vi "Module Information.vi"(7 "Module Name":string="Module") -> ()   [LabVIEW 2017, in "DebugConsole.lvlib"]
uses:
  DebugConsole.lvlib
  _Support/Typedef/_CSM_MODE.ctl
  _Support/CSMQ/_CSMOFGVOPER.ctl
  _csmlite/_PassAllowedMessage - MsgList.vi
  _csmlite/_csmlite.lvlib
  Communicable State Machine.lvlib
  _ui/csm-ui-support.lvlib
panel:
  in  "CSM":string
  out "#Nodes":i32
  out "Mode":T1=enum."Stand Alone"
  out "inlvlibp":bool
  out "interStop":bool
  out "#Elements In Queue":i32
  out "Initialized":enum16{"Initializing", "Ready", "Exiting"}(ring)
  out "RemoteMessge?":bool
  out "Current State":string
  out "Remaing States":string
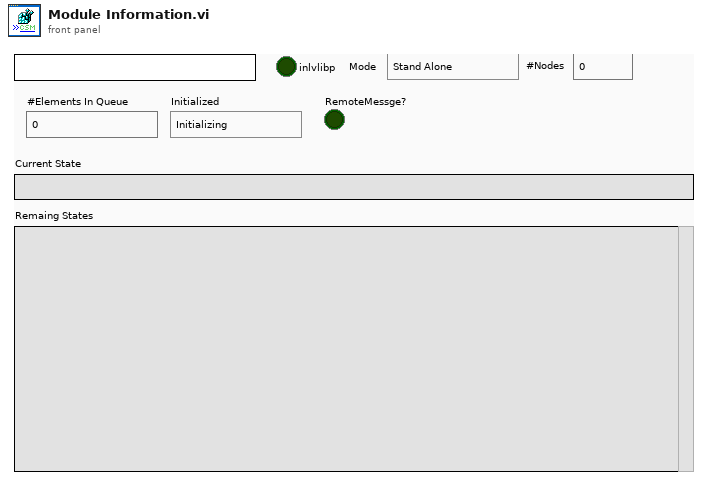
[diagram p1: front panel]
types:
  T1 = typedef "Communicable State Machine.lvlib/_CSM_MODE.ctl" = enum16{"Not Exist", "Stand Alone", "CSM", "Worker", "Worker Agent", "Chain Node", "Chain"}
  T2 = enum32{"Invalid", "Standard", "Closed", "Hidden", "Minimized", "Maximized"}
  T3 = enum32{"invalid app kind", "Development System", "Run Time System", "Student Edition", "Embedded LabVIEW", "Evaluation", "Custom"}
  T4 = cluster{"Core":cluster{"Current VI Reference":refnum<vi>, "Close Panel on Exit?":bool}, "Your Boolean data":bool, "Your string data":string}
  T5 = cluster{"Current VI Reference":refnum<vi>, "Close Panel on Exit?":bool}
  T6 = typedef "Communicable State Machine.lvlib/_CSMOFGVOPER.ctl" = enum16{"Create If not Exist", "Get By Name", "List", "Check If Name Exists", "Release", "Module Status", "Create Status Event Handler", "Destroy Status Event Handler", "Clear Invalid Objs"}
  T7 = enum8{"Enabled", "Disabled", "Disabled and Grayed Out"}
  T8 = typedef "Communicable State Machine.lvlib/_CSMObj.ctl" = cluster{"info":T9, "Refs":T10}
  T9 = typedef "Communicable State Machine.lvlib/_CSMObj-Info.ctl" = cluster{"Module Name":string, "Requested Name":string, "Group Name":string, "Mode":T1, "Allowed Messages":string[]}
  T10 = typedef "Communicable State Machine.lvlib/_CSMObj-Refs.ctl" = cluster{"WatchDogQ":refnum<queue>, "CSMDataDVR":refnum<data-value>, "Queue":T11, "GroupDataDVR":refnum<data-value>, "TagMap":refnum<data-value>, "ExitEvent":refnum<user-event>, "NewStateEvent":refnum<user-event>, "StatusEvent":refnum<user-event>, "InterruptEvent":refnum<user-event>}
  T11 = typedef "Communicable State Machine.lvlib/Priority Queue.ctl" = cluster{"HPriorityQ":refnum<queue>, "LowPriorityQ":refnum<queue>}
  T12 = typedef "Communicable State Machine.lvlib/_CSMObj-Data.ctl" = cluster{"RemoteMessge?":bool, "error":errorcluster, "Return State":string, "Initialized":enum16{"Initializing", "Ready", "Exiting"}, "InternalRegistryRules":string[], "Return Msg Type":T13, "Current State":string, "Remaing JKISM Queue":string}
  T13 = typedef "Communicable State Machine.lvlib/_CSM_MSG_TYPE.ctl" = enum16{"Sync Message(-@)", "Async Message(->)", "Async without Response(->|)", "Async Response", "Broadcast(-><all>)", "Broadcast(-><status>)", "Broadcast(-><interrupt>)", "Append to JKISM States", "Append to JKISM States(High Priority)", "Broadcast(-><state>)", "<None>"}
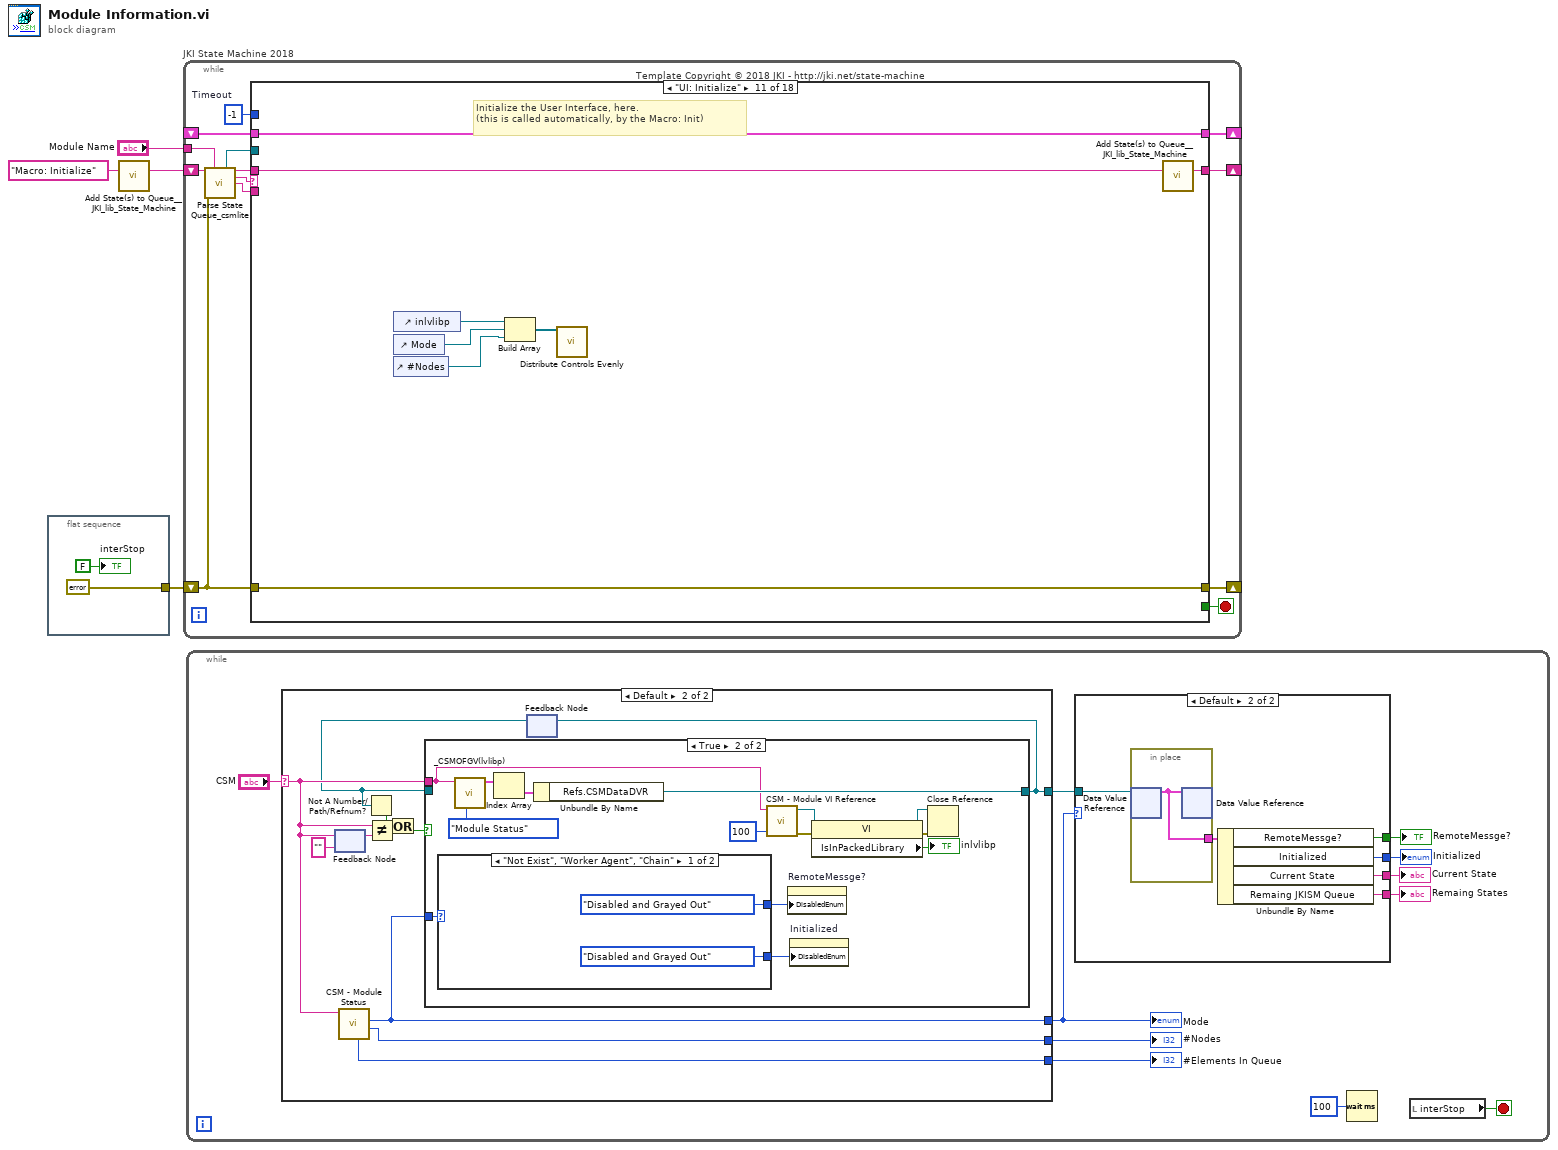
[diagram p0: block diagram]
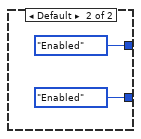
[diagram p5: hidden frame]
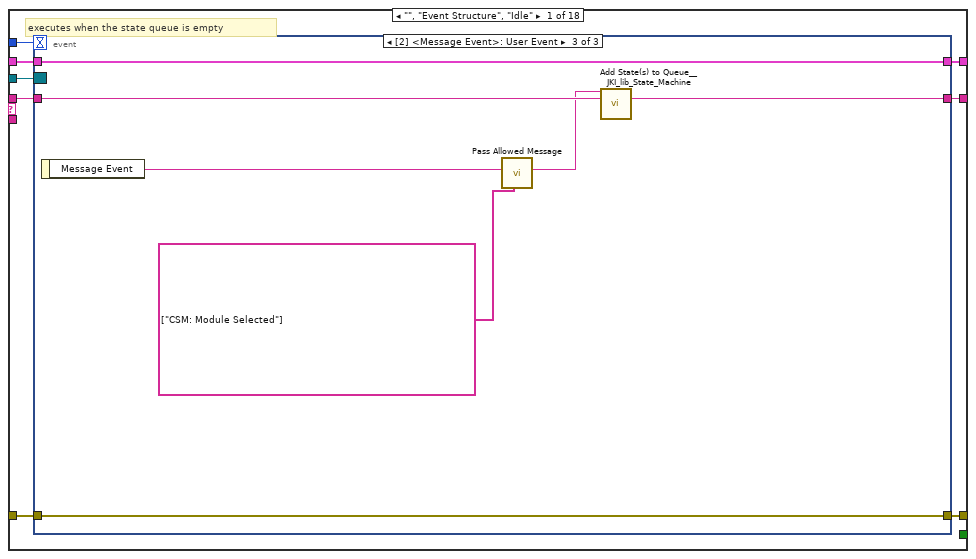
[diagram p6: hidden frame]
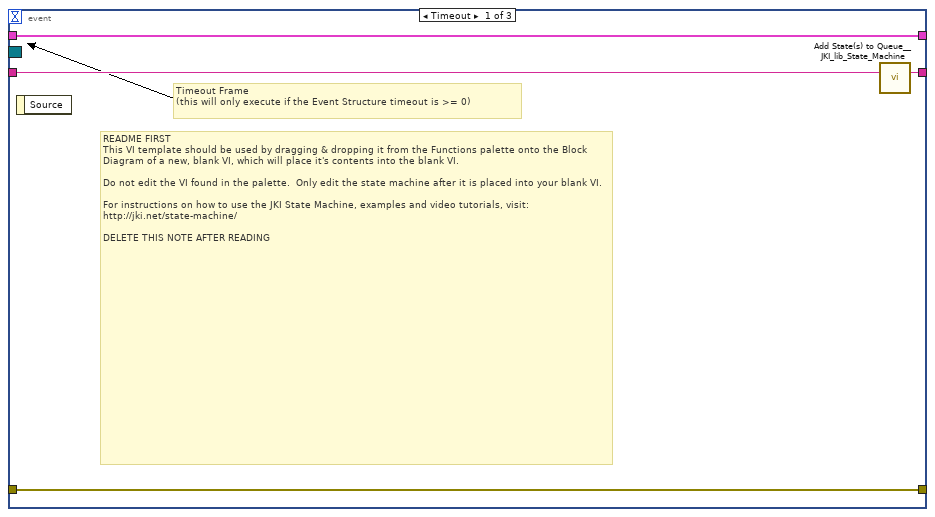
[diagram p7: hidden frame]
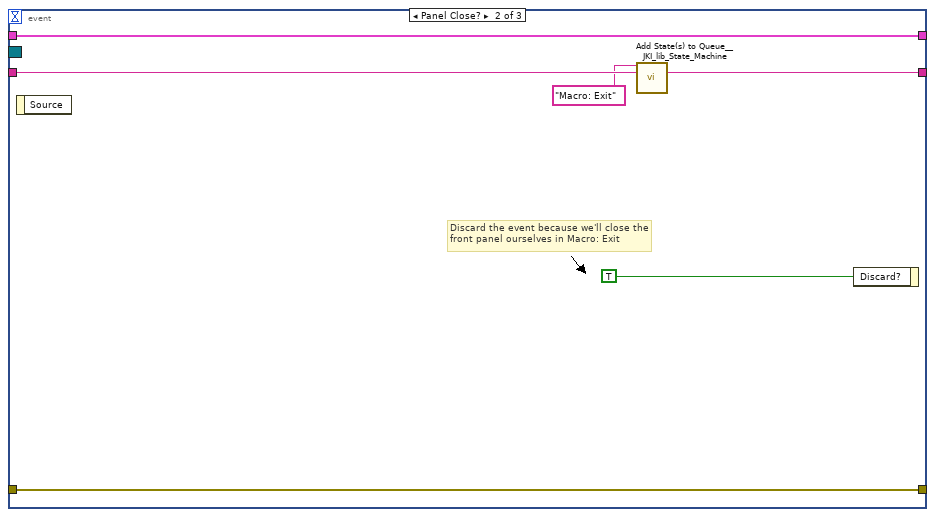
[diagram p8: hidden frame]
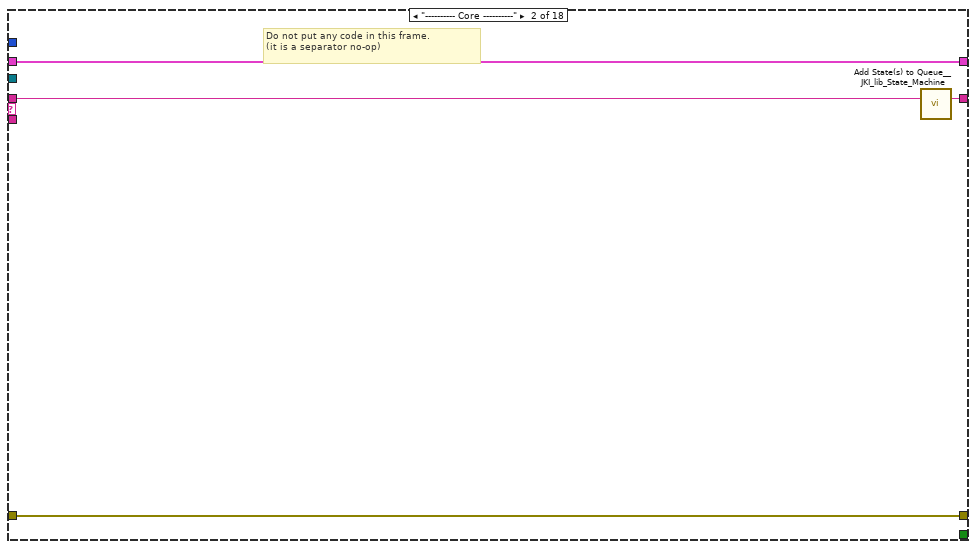
[diagram p9: hidden frame]
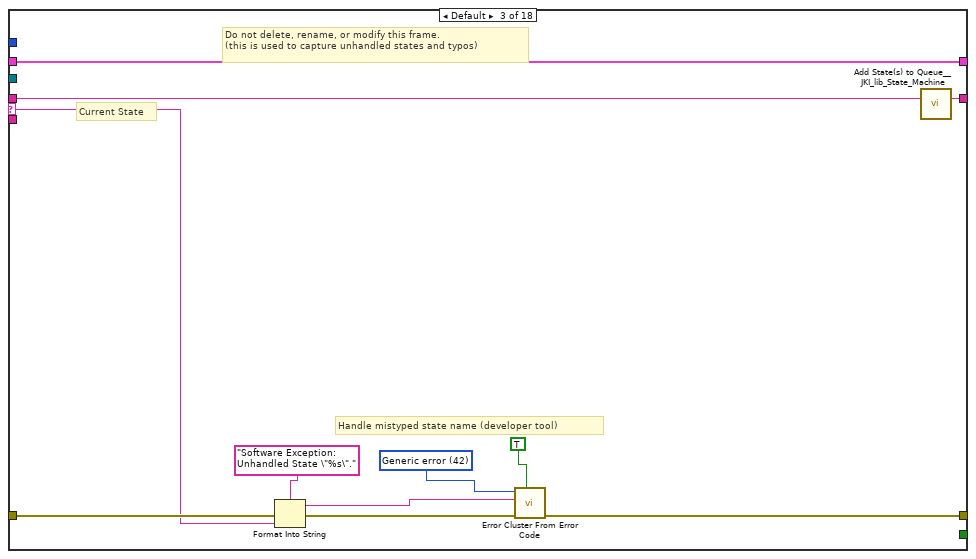
[diagram p10: hidden frame]
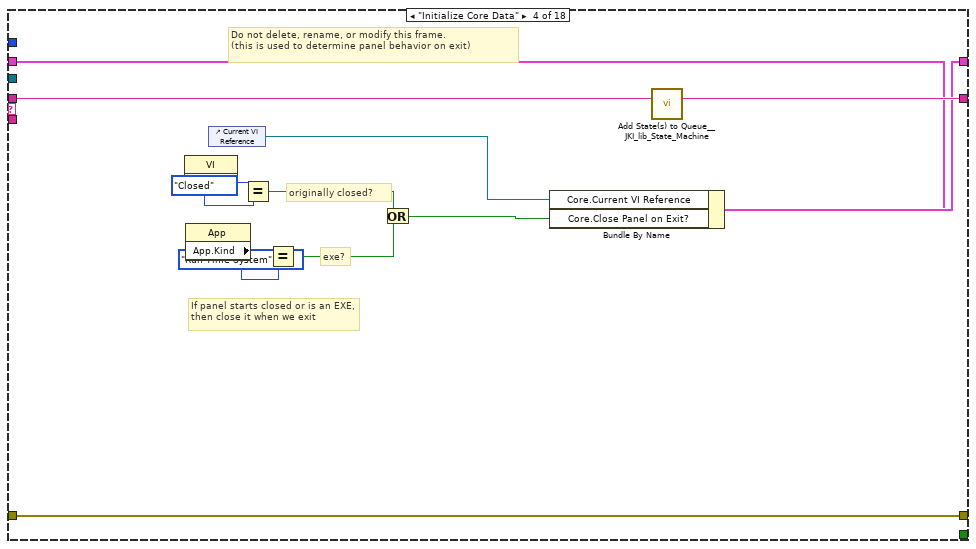
[diagram p11: hidden frame]
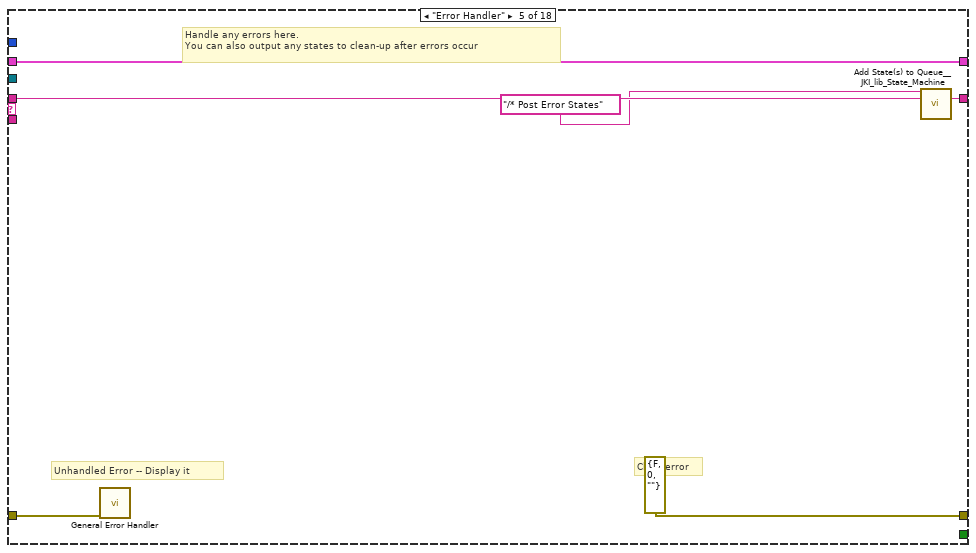
[diagram p12: hidden frame]
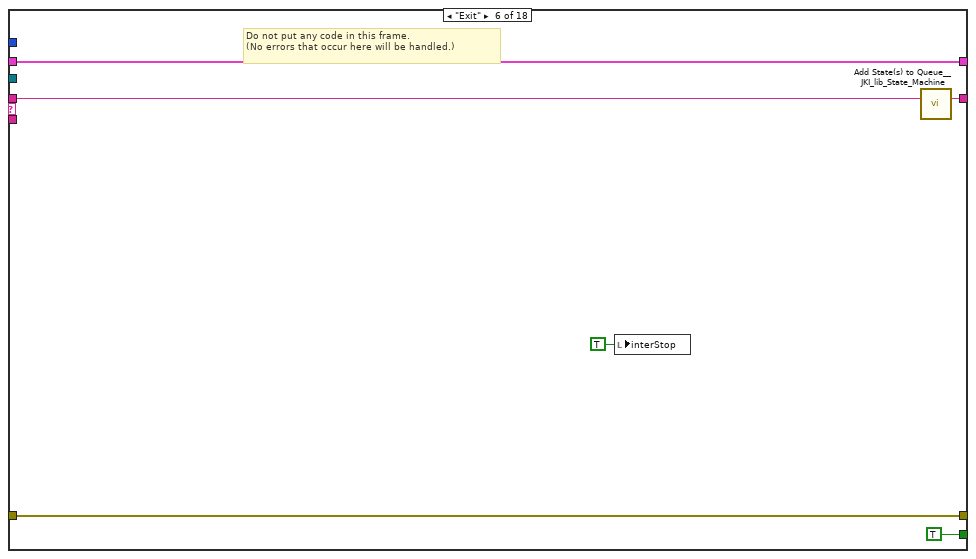
[diagram p13: hidden frame]
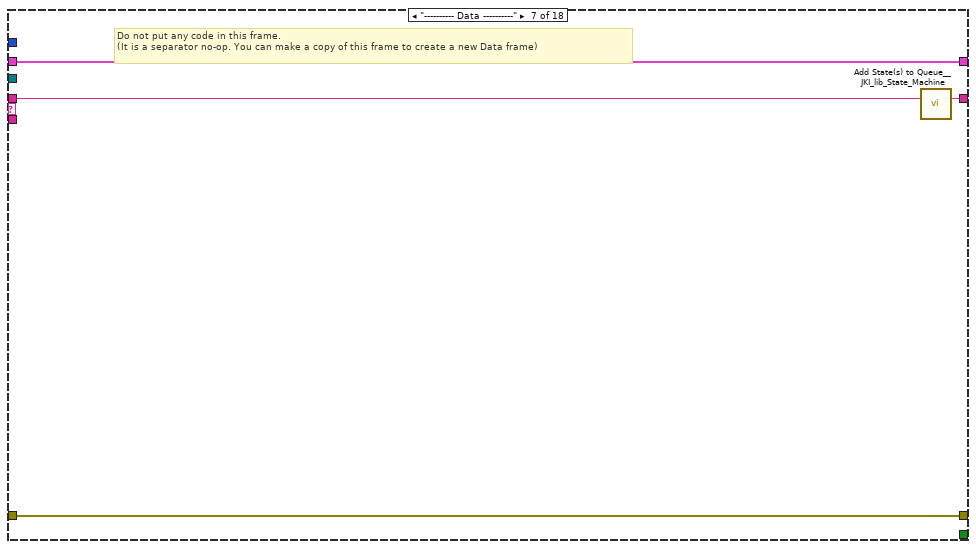
[diagram p14: hidden frame]
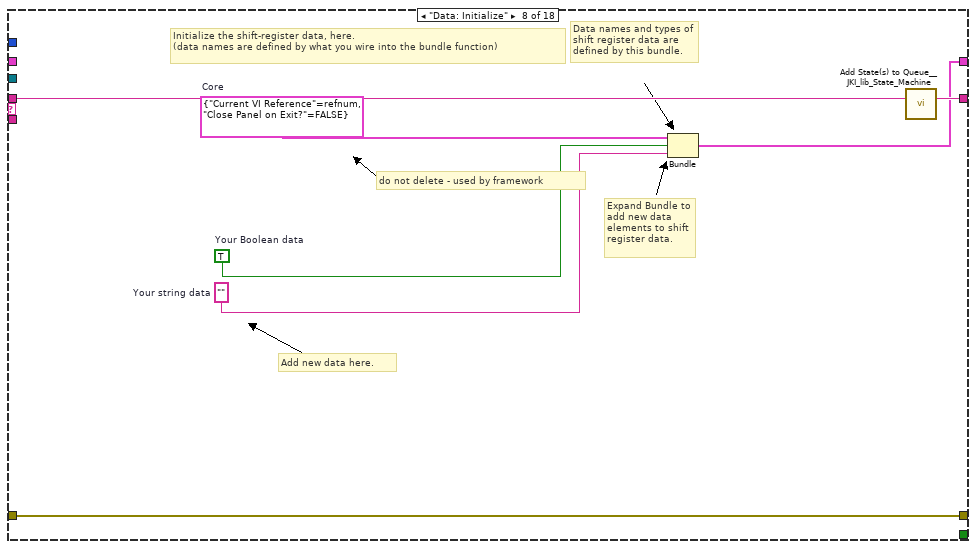
[diagram p15: hidden frame]
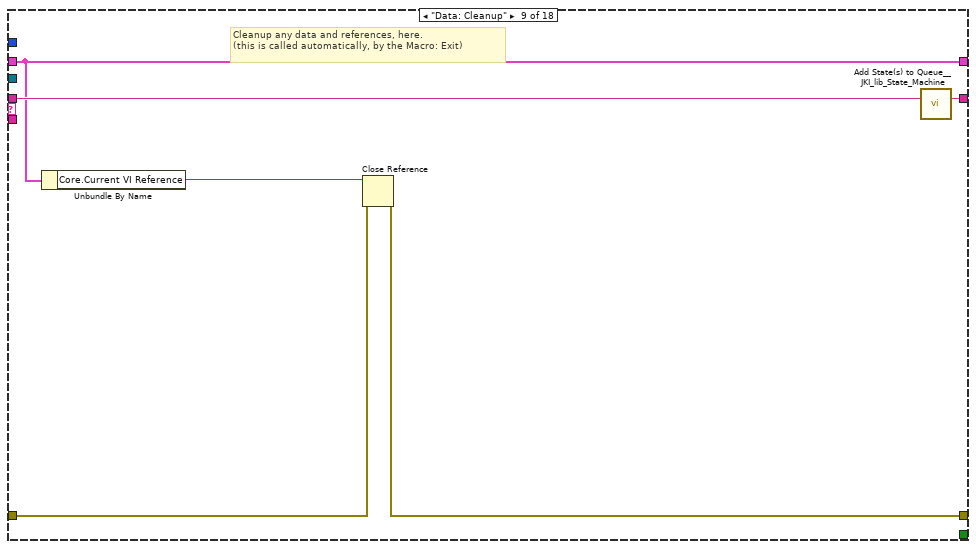
[diagram p16: hidden frame]
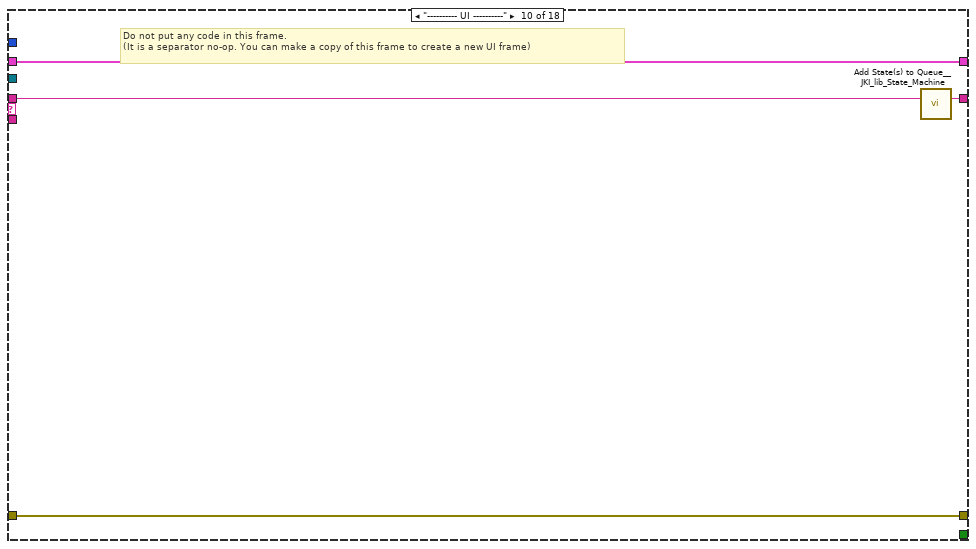
[diagram p17: hidden frame]
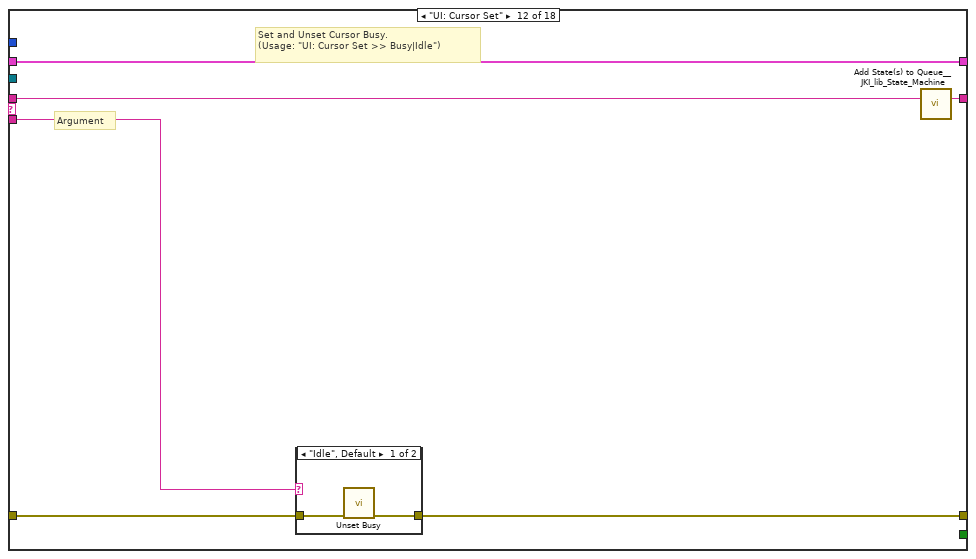
[diagram p18: hidden frame]
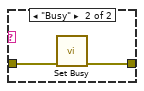
[diagram p19: hidden frame]
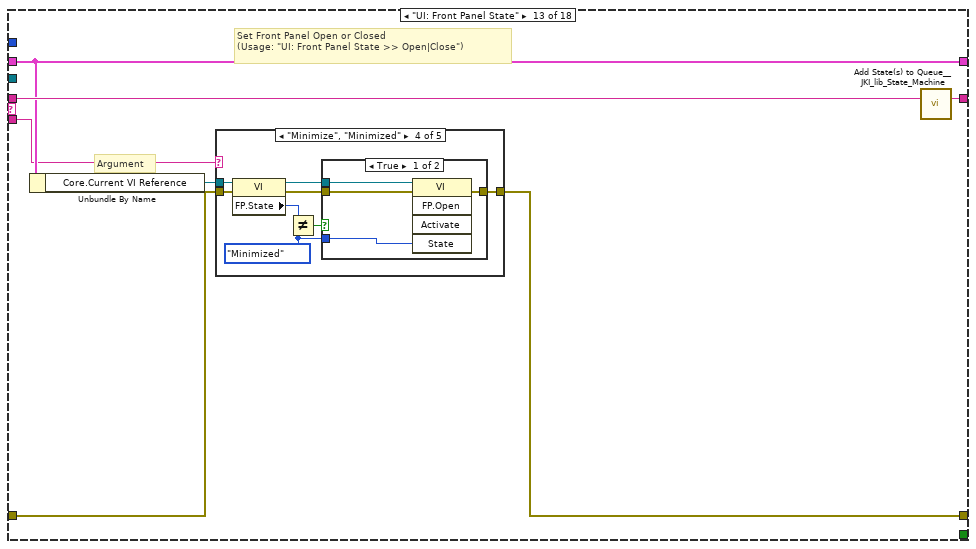
[diagram p20: hidden frame]
diagram:
  n1 = flat-sequence {
    tunnel: [errorcluster {"status"=FALSE, "code"=0, "source"=""} ("error out")] -> w1
    frame #0 {
      "interStop" <- FALSE ("Boolean")
    }
  }
  n2 = call <vilib>:"Add State(s) to Queue__JKI_lib_State_Machine.vi"("State(s) in (\"\")"="Macro: Initialize") -> ("States Out"=w3:string)  [unwired: 14 in]
  n3 = while "JKI State Machine 2018" {
    shift-right: [w12] -> _
    shift-left: _ -> [w11]
    shift-right: [w15] -> _
    shift-left: w1 -> [w9]
    shift-right: [w14] -> _
    shift-left: w3 -> [w16]
    tunnel: "Module Name" -> [w8]
    stop <- w13 stop-if-true
    w10 = -1  # Timeout
    # "Template Copyright © 2018 JKI - http://jki.net/state-machine"
    n4 = call "Parse State Queue_csmlite.vi"("State Queue"=w16, "Current Module(\"\" to generate an ID)"=w8, "Error In (no error)"=w9) -> ("Event Registration Refnum"=w7:refnum<event-registration>, "Remaining States"=w18:string, "Current State"=w19:string, "Arguments"=w17:string)  [unwired: 9 in]
    n5 = case shown="\"UI: Initialize\"" w19 {
      selector: w19 -> [_ _ w49 _ _ _ _ _ _ _ _ _ _ _ _ _ _ _]
      tunnel: w18 -> [w27 w48 w53 w72 w78 w84 w88 w95 w101 w105 w113 w119 w130 w199 w204 w214 w218 w221]
      tunnel: w17 -> [_ _ _ _ _ _ _ _ _ _ _ w114 w124 _ _ _ _ w219]
      tunnel: w11 -> [w25 w45 w51 w65 w75 w82 w85 _ w96 w102 w111 w117 w126 w196 w201 w211 w215 w220]
      tunnel: [w24 w46 w55 w69 errorcluster {"status"=FALSE, "code"=0, "source"=""} ("error out") w81 w86 w92 w97 w103 w110 w115 w127 w197 w202 w212 w216 w222] -> w15
      tunnel: w9 -> [w23 w46 w54 w69 w74 w81 w86 w92 w98 w103 w110 w116 w128 w197 w202 w212 w216 w222]
      tunnel: [w26 w47 w52 w71 w77 w83 w87 w94 w100 w104 w112 w118 w129 w198 w203 w213 w217 w221] -> w14
      tunnel: [_ _ _ _ _ TRUE _ _ _ _ _ _ _ _ _ _ _ _] -> w13
      tunnel: [w22 w45 w51 w70 w75 w82 w85 w93 w96 w102 w111 w117 w126 w196 w201 w211 w215 w220] -> w12
      tunnel: w10 -> [w21 _ _ _ _ _ _ _ _ _ _ _ _ _ _ _ _ _]
      tunnel: w7 -> [w20 _ _ _ _ _ _ _ _ _ _ _ _ _ _ _ _ _]
      frame "", "Event Structure", "Idle" {
        # "executes when the state queue is empty"
        n6 = event shown="[2] <Message Event>: User Event" {
          selector: w20 -> [_ _ _]
          dyn-events: _ -> [_ _ _]
          timeout: w21 -> [_ _ _]
          tunnel: w27 -> [w31 w37 w42]
          tunnel: [w30 w36 w40] -> w26
          tunnel: w25 -> [w28 w34 w43]
          tunnel: [w29 w35 w44] -> w24
          tunnel: w23 -> [w29 w35 w44]
          tunnel: [w28 w34 w43] -> w22
          event Timeout {
            # "README FIRST\nThis VI template should be used by dragging & dropping it from the Functions palette onto the Block Diagram of a new, blank VI, which will place it's contents into the blank VI.\n\nDo not edit the VI found in the palette.  Only edit the state machine after it is placed into your blank VI.\n\nFor instructions on how to use the JKI State Machine, examples and video tutorials, visit:\nhttp://jki.net/state-machine/\n\nDELETE THIS NOTE AFTER READING"
            # "Timeout Frame\n(this will only execute if the Event Structure timeout is >= 0)"
            n7 = event-data() -> ()  [unwired: 1 in, 1 out]
            n8 = call <vilib>:"Add State(s) to Queue__JKI_lib_State_Machine.vi"("State(s) in (\"\")"=w31) -> ("States Out"=w30:string)  [unwired: 14 in]
          }
          event Panel Close? {
            # "Discard the event because we'll close the front panel ourselves in Macro: Exit"
            n9 = event-data() -> ()  [unwired: 1 in, 1 out]
            n10 = call <vilib>:"Add State(s) to Queue__JKI_lib_State_Machine.vi"("State(s) in Front (\"\")"="Macro: Exit", "State(s) in (\"\")"=w37) -> ("States Out"=w36:string)  [unwired: 13 in]
            n11 = event-data("Discard?"=TRUE) -> ()  [unwired: 1 in, 1 out]
          }
          event User Event {
            n12 = event-data() -> ("Message Event"=w41:string)  [unwired: 1 in]
            n13 = call-poly "Pass Allowed Message.vi"("Allowed Message"=string[] ["CSM: Module Selected"], "JKISM External Event"=w41) -> ("States"=w39:string)  [unwired: 7 in]
            n14 = call <vilib>:"Add State(s) to Queue__JKI_lib_State_Machine.vi"("State(s) in Front (\"\")"=w39, "State(s) in (\"\")"=w42) -> ("States Out"=w40:string)  [unwired: 13 in]
          }
        }
      }
      frame "---------- Core ----------" {
        # "Do not put any code in this frame.\n(it is a separator no-op)"
        n15 = call <vilib>:"Add State(s) to Queue__JKI_lib_State_Machine.vi"("State(s) in (\"\")"=w48) -> ("States Out"=w47:string)  [unwired: 14 in]
      }
      frame Default {
        w58 = 42 items=["No error", "Argument error", "Memory is full", "Out of zone", "End of file", "File already open", "Generic file I/O error", "File not found", "File permission error", "Disk is full", "Duplicate path", "Too many files open", "System feature not enabled", "Resource file not found", "Cannot add resource", "Resource not found", "Image not found", "Image memory error", "Pen does not exist", "Config type invalid", "Config token not found", "Config parse error", "Config memory error", "Bad external code format", "Bad external code offset", "External code not present", "Null window", "Destroy window error", "Null menu", "Print aborted", "Bad print record", "Print driver error", "Windows error during printing", "Memory error during printing", "Print dialog error", "Generic print error", "Invalid device refnum", "Device not found", "Device parameter error", "Device unit error", "Cannot open device", "Device call aborted", "Generic error", "Cancelled by user", "Object ID too low", "Object ID too high", "Object not in heap", "Unknown heap", "Unknown object (invalid DefProc)", "Unknown object (DefProc not in table)", "Message out of range", "Invalid (null) method", "Unknown message", "Manager call not supported", "Bad address", "Network operation in progress", "Network operation timed out", "Connection is busy", "Network attribute not supported", "Network error", "Address in use", "System out of memory", "Connection aborted", "Connection refused", "Not connected", "Already connected", "Connection closed", "Initialization error (interapplication manager)", "Bad occurrence", "Wait on unbound occurrence handler", "Occurrence queue overflow", "Datalog type conflict", "Unused", "Unrecognized type (interapplication manager)", "Memory corrupt", "Failed to make temporary DLL", "Old CIN version", "Drag socket not found", "Failed to load drop-object", "Failed to register OLE object", "Failed to release OLE object", "Format specifier type mismatch", "Unknown format specifier", "Too few format specifiers", "Too many format specifiers", "Scan failed", "Newer CIN version", "Error converting to variant", "Runtime menu error", "Password tampered", "Variant attribute not found", "Incompatible variant data type", "Event data is not available", "Event Store is not present", "Occurrence is not found", "Event Queue is not created", "Event info is not available", "Refnum passed is NULL", "Error retrieving Class GUID", "Error retrieving CoClass GUID", "Error retrieving TypeLib GUID.", "Bad built application magic bytes.", "Specific driver is different from the specific driver associated with the Logical Name.", "There is no session opened to the class driver.", "Max Error", "MAX - Error with config objects", "MAX - Error loading configuration", "MAX - Group not supported"]
        # "Current State"
        # "Do not delete, rename, or modify this frame.\n(this is used to capture unhandled states and typos)"
        # "Handle mistyped state name (developer tool)"
        n16 = Format Into String(format string="Software Exception: Unhandled State \"%s\"." ("message"), error in=w54, w49) -> (resulting string=w57:string, error out=w56:errorcluster)  [unwired: 1 in]
        n17 = call <vilib>:"Error Cluster From Error Code.vi"("show call chain? (False)"=TRUE, "error in (no error)"=w56, "error message (\"\")"=w57, "error code (0)"=w58) -> ("error out"=w55:errorcluster)  [unwired: 5 in]
        n18 = call <vilib>:"Add State(s) to Queue__JKI_lib_State_Machine.vi"("State(s) in (\"\")"=w53) -> ("States Out"=w52:string)  [unwired: 14 in]
      }
      frame "Initialize Core Data" {
        # "Do not delete, rename, or modify this frame.\n(this is used to determine panel behavior on exit)"
        # "originally closed?"
        # "exe?"
        # "If panel starts closed or is an EXE, then close it when we exit"
        n19 = property class="VI"() -> ("FP.State"=w62:T2)  [unwired: 2 in, 2 out]
        n20 = property class="App"() -> ("App.Kind"=w68:T3)  [unwired: 2 in, 2 out]
        n21 = control-ref of="Current VI Reference"() -> (w63:refnum<vi>)
        n22 = Equal?(x=w62, y=T2."Closed" ("Front Panel Window:State")) -> (x = y?=w60:bool)
        n23 = Equal?(x=w68, y=T3."Run Time System" ("Application:Kind")) -> (x = y?=w66:bool)
        n24 = Or(x=w60, y=w66) -> (x .or. y?=w64:bool)
        n25 = Bundle By Name(cluster=w65, "Core.Current VI Reference"=w63, "Core.Close Panel on Exit?"=w64) -> (w70:T4)
        n26 = call <vilib>:"Add State(s) to Queue__JKI_lib_State_Machine.vi"("State(s) in (\"\")"=w72) -> ("States Out"=w71:string)  [unwired: 14 in]
      }
      frame "Error Handler" {
        # "Unhandled Error -- Display it"
        # "Handle any errors here.\nYou can also output any states to clean-up after errors occur"
        # "Clear error"
        n27 = call <vilib>:"General Error Handler.vi"("error in (no error)"=w74) -> ()  [unwired: 10 in, 5 out]
        n28 = call <vilib>:"Add State(s) to Queue__JKI_lib_State_Machine.vi"("State(s) in Front (\"\")"="/* Post Error States", "State(s) in (\"\")"=w78) -> ("States Out"=w77:string)  [unwired: 13 in]
      }
      frame "Exit" {
        # "Do not put any code in this frame.\n(No errors that occur here will be handled.)"
        n29 = local write "interStop"(TRUE ("interStop")) -> ()
        n30 = call <vilib>:"Add State(s) to Queue__JKI_lib_State_Machine.vi"("State(s) in (\"\")"=w84) -> ("States Out"=w83:string)  [unwired: 14 in]
      }
      frame "---------- Data ----------" {
        # "Do not put any code in this frame.\n(It is a separator no-op. You can make a copy of this frame to create a new Data frame)"
        n31 = call <vilib>:"Add State(s) to Queue__JKI_lib_State_Machine.vi"("State(s) in (\"\")"=w88) -> ("States Out"=w87:string)  [unwired: 14 in]
      }
      frame "Data: Initialize" {
        w89 = T5 {"Current VI Reference"=refnum, "Close Panel on Exit?"=FALSE}  # Core
        w91 = TRUE  # Your Boolean data
        w90 = ""  # Your string data
        # "do not delete - used by framework"
        # "Expand Bundle to add new data elements to shift register data."
        # "Add new data here."
        # "Data names and types of shift register data are defined by this bundle."
        # "Initialize the shift-register data, here.\n(data names are defined by what you wire into the bundle function)"
        n32 = Bundle("Core"=w89, "Your Boolean data"=w91, "Your string data"=w90) -> (w93:T4)  [unwired: 1 in]
        n33 = call <vilib>:"Add State(s) to Queue__JKI_lib_State_Machine.vi"("State(s) in (\"\")"=w95) -> ("States Out"=w94:string)  [unwired: 14 in]
      }
      frame "Data: Cleanup" {
        # "Cleanup any data and references, here.\n(this is called automatically, by the Macro: Exit)"
        n34 = Unbundle By Name(w96) -> ("Core.Current VI Reference"=w99:refnum<vi>)
        n35 = Close Reference(reference=w99, error in (no error)=w98) -> (error out=w97:errorcluster)
        n36 = call <vilib>:"Add State(s) to Queue__JKI_lib_State_Machine.vi"("State(s) in (\"\")"=w101) -> ("States Out"=w100:string)  [unwired: 14 in]
      }
      frame "---------- UI ----------" {
        # "Do not put any code in this frame.\n(It is a separator no-op. You can make a copy of this frame to create a new UI frame)"
        n37 = call <vilib>:"Add State(s) to Queue__JKI_lib_State_Machine.vi"("State(s) in (\"\")"=w105) -> ("States Out"=w104:string)  [unwired: 14 in]
      }
      frame "UI: Initialize" {
        # "Initialize the User Interface, here.\n(this is called automatically, by the Macro: Init)"
        n38 = control-ref of="inlvlibp"() -> (w106:refnum<vi>)
        n39 = control-ref of="Mode"() -> (w107:refnum<vi>)
        n40 = control-ref of="#Nodes"() -> (w108:refnum<vi>)
        n41 = Build Array(w106, w107, w108) -> (w109:refnum<vi>[])
        n42 = call "Distribute Controls Evenly.vi"("Controls"=w109) -> ()  [unwired: 10 in, 1 out]
        n43 = call <vilib>:"Add State(s) to Queue__JKI_lib_State_Machine.vi"("State(s) in (\"\")"=w113) -> ("States Out"=w112:string)  [unwired: 14 in]
      }
      frame "UI: Cursor Set" {
        # "Argument"
        # "Set and Unset Cursor Busy.\n(Usage: \"UI: Cursor Set >> Busy|Idle\")"
        n44 = case shown="\"Idle\", Default" w114 {
          tunnel: w116 -> [w121 w123]
          tunnel: [w120 w122] -> w115
          frame "Idle", Default {
            n45 = call <vilib>:"Unset Busy.vi"("error in (no error)"=w121) -> ("error out"=w120:errorcluster)  [unwired: 10 in]
          }
          frame "Busy" {
            n46 = call <vilib>:"Set Busy.vi"("error in (no error)"=w123) -> ("error out"=w122:errorcluster)  [unwired: 9 in, 1 out]
          }
        }
        n47 = call <vilib>:"Add State(s) to Queue__JKI_lib_State_Machine.vi"("State(s) in (\"\")"=w119) -> ("States Out"=w118:string)  [unwired: 14 in]
      }
      frame "UI: Front Panel State" {
        # "Argument"
        # "Set Front Panel Open or Closed\n(Usage: \"UI: Front Panel State >> Open|Close\")"
        n48 = Unbundle By Name(w126) -> ("Core.Current VI Reference"=w125:refnum<vi>)
        n49 = case shown="\"Minimize\", \"Minimized\"" w124 {
          tunnel: w128 -> [w136 w151 w162 w175 w188]
          tunnel: [w138 w152 w164 w177 w190] -> w127
          tunnel: w125 -> [w137 w149 w163 w176 w189]
          frame "Open", "Standard", Default {
            w131 = T2."Standard" ("State")
            n50 = property class="VI"(reference=w137, error in=w136) -> (reference out=w134:refnum<vi>, error out=w135:errorcluster, "FP.State"=w133:T2)
            n51 = Not Equal?(x=w133, y=w131) -> (x != y?=w132:bool)
            n52 = case shown="True" w132 {
              tunnel: [w142 w144] -> w138
              tunnel: w135 -> [w141 w144]
              tunnel: w134 -> [w140 _]
              tunnel: w131 -> [w139 _]
              frame True {
                n53 = invoke class="VI" method="FP.Open"(reference=w140, error in=w141, "Activate"=TRUE, "State"=w139) -> (error out=w142:errorcluster)  [unwired: 1 in, 4 out]
              }
              frame False {
              }
            }
          }
          frame "Close", "Closed" {
            n54 = property class="VI"(reference=w149, error in=w151) -> (reference out=w148:refnum<vi>, error out=w150:errorcluster, "FP.State"=w146:T2)
            n55 = Not Equal?(x=w146, y=T2."Closed" ("Front Panel Window:State")) -> (x != y?=w145:bool)
            n56 = case shown="True" w145 {
              tunnel: [w153 w156] -> w152
              tunnel: w150 -> [w153 w155]
              tunnel: w148 -> [_ w154]
              frame False {
              }
              frame True {
                n57 = invoke class="VI" method="FP.Close"(reference=w154, error in=w155) -> (error out=w156:errorcluster)  [unwired: 1 in, 2 out]
              }
            }
          }
          frame "Hidden", "Hide" {
            w157 = T2."Hidden" ("State")
            n58 = property class="VI"(reference=w163, error in=w162) -> (reference out=w160:refnum<vi>, error out=w161:errorcluster, "FP.State"=w159:T2)
            n59 = Not Equal?(x=w159, y=w157) -> (x != y?=w158:bool)
            n60 = case shown="True" w158 {
              tunnel: [w168 w169] -> w164
              tunnel: w161 -> [w167 w169]
              tunnel: w160 -> [w166 _]
              tunnel: w157 -> [w165 _]
              frame True {
                n61 = invoke class="VI" method="FP.Open"(reference=w166, error in=w167, "State"=w165) -> (error out=w168:errorcluster)  [unwired: 2 in, 4 out]
              }
              frame False {
              }
            }
          }
          frame "Minimize", "Minimized" {
            w170 = T2."Minimized" ("State")
            n62 = property class="VI"(reference=w176, error in=w175) -> (reference out=w173:refnum<vi>, error out=w174:errorcluster, "FP.State"=w172:T2)
            n63 = Not Equal?(x=w172, y=w170) -> (x != y?=w171:bool)
            n64 = case shown="True" w171 {
              tunnel: [w181 w182] -> w177
              tunnel: w174 -> [w180 w182]
              tunnel: w173 -> [w179 _]
              tunnel: w170 -> [w178 _]
              frame True {
                n65 = invoke class="VI" method="FP.Open"(reference=w179, error in=w180, "State"=w178) -> (error out=w181:errorcluster)  [unwired: 2 in, 4 out]
              }
              frame False {
              }
            }
          }
          frame "Maximize", "Maximized" {
            w183 = T2."Maximized" ("State")
            n66 = property class="VI"(reference=w189, error in=w188) -> (reference out=w186:refnum<vi>, error out=w187:errorcluster, "FP.State"=w185:T2)
            n67 = Not Equal?(x=w185, y=w183) -> (x != y?=w184:bool)
            n68 = case shown="True" w184 {
              tunnel: [w194 w195] -> w190
              tunnel: w187 -> [w193 w195]
              tunnel: w186 -> [w192 _]
              tunnel: w183 -> [w191 _]
              frame True {
                n69 = invoke class="VI" method="FP.Open"(reference=w192, error in=w193, "State"=w191) -> (error out=w194:errorcluster)  [unwired: 2 in, 4 out]
              }
              frame False {
              }
            }
          }
        }
        n70 = call <vilib>:"Add State(s) to Queue__JKI_lib_State_Machine.vi"("State(s) in (\"\")"=w130) -> ("States Out"=w129:string)  [unwired: 14 in]
      }
      frame "---------- Macro ----------" {
        # "Do not put any code in this frame.\n(It is a separator no-op. You can make a copy of this frame to create a new Macro frame)"
        n71 = call <vilib>:"Add State(s) to Queue__JKI_lib_State_Machine.vi"("State(s) in (\"\")"=w199) -> ("States Out"=w198:string)  [unwired: 14 in]
      }
      frame "Macro: Initialize" {
        # "Initialization Macro\n(This is called once, when the VI starts)"
        n72 = call <vilib>:"Add State(s) to Queue__JKI_lib_State_Machine.vi"("State(s) in Front (\"\")"="Data: Initialize\nInitialize Core Data\nUI: Initialize", "State(s) in (\"\")"=w204) -> ("States Out"=w203:string)  [unwired: 13 in]
      }
      frame "Macro: Exit" {
        # "Exit Macro\n(This is called once, when the VI exits)"
        n73 = Unbundle By Name(w211) -> ("Core.Close Panel on Exit?"=w210:bool)
        n74 = Select(t="//UI: Front Panel State >> Close", s=w210, f="") -> (s? t:f=w207:string)
        n75 = call <vilib>:"Add State(s) to Queue__JKI_lib_State_Machine.vi"("State(s) in (\"\")"=w207, "State(s) at Back (\"\")"="Data: Cleanup\nExit") -> ("States Out"=w205:string)  [unwired: 13 in]
        n76 = call <vilib>:"Add State(s) to Queue__JKI_lib_State_Machine.vi"("State(s) in Front (\"\")"=w205, "State(s) in (\"\")"=w214) -> ("States Out"=w213:string)  [unwired: 13 in]
      }
      frame "---------- Action ----------" {
        n77 = call <vilib>:"Add State(s) to Queue__JKI_lib_State_Machine.vi"("State(s) in (\"\")"=w218) -> ("States Out"=w217:string)  [unwired: 14 in]
      }
      frame "CSM: Module Selected" {
        n78 = local write "CSM"(w219) -> ()
      }
    }
  }
  n79 = while {
    stop <- w232 stop-if-true
    n80 = case shown="Default" "CSM" {
      selector: "CSM" -> [_ w249]
      tunnel: [_ w246] -> w233
      tunnel: [_ w244] -> w225
      tunnel: [_ w251] -> w227
      tunnel: [_ w250] -> w226
      frame "" {
      }
      frame Default {
        n81 = feedback-in #1(w249) -> ()
        n82 = feedback #1("") -> (w248:string)
        n83 = call "CSM - Module Status.vi"("CSM Name"=w249) -> ("#Nodes"=w251:i32, "Mode"=w244:T1, "#Elements In Queue"=w250:i32)  [unwired: 6 in, 2 out]
        n84 = Not Equal?(x=w249, y=w248) -> (x != y?=w245:bool)
        n85 = feedback #2() -> (w241:refnum<data-value>)  [unwired: 1 in]
        n86 = Not A Number/Path/Refnum?(number/path/refnum=w241) -> (NaN/Path/Refnum?=w242:bool)
        n87 = Or(x=w242, y=w245) -> (x .or. y?=w243:bool)
        n88 = case shown="True" w243 {
          tunnel: [w252 w263] -> w246
          tunnel: w249 -> [_ w253]
          tunnel: w241 -> [w252 _]
          tunnel: w244 -> [_ w262]
          frame False {
          }
          frame True {
            n89 = case shown="\"Not Exist\", \"Worker Agent\", \"Chain\"" w262 {
              tunnel: [T7."Disabled and Grayed Out" ("Disabled") T7."Enabled" ("Disabled")] -> w261
              tunnel: [T7."Disabled and Grayed Out" ("Disabled") T7."Enabled" ("Disabled")] -> w260
              frame "Not Exist", "Worker Agent", "Chain" {
              }
              frame Default {
              }
            }
            n90 = call "_CSMOFGV(lvlibp).vi"("Operation"=_CSMOFGVOPER."Module Status", "Name (\"\" to Use UUID) In"=w253) -> ("Array"=w265:T8[])  [unwired: 7 in, 2 out]
            n91 = Index Array(array=w265) -> (element=w266:T8)  [unwired: 1 in]
            n92 = Unbundle By Name(w266) -> ("Refs.CSMDataDVR"=w263:refnum<data-value>)
            n93 = call "CSM - Module VI Reference.vi"("Response Timeout (-2 Using Global Settings)"=100 ("Response Timeout(5000 ms)"), "CSM Name"=w253) -> ("error out"=w256:errorcluster, "CSM Module VIRef"=w255:refnum<vi>)  [unwired: 8 in]
            n94 = property on="RemoteMessge?" class="Bool (strict)"("DisabledEnum"=w260) -> ()  [unwired: 2 in, 2 out]
            n95 = property on="Initialized" class="Enum (strict)"("DisabledEnum"=w261) -> ()  [unwired: 2 in, 2 out]
            n96 = property class="VI"(reference=w255, error in=w256) -> (reference out=w257:refnum<vi>, error out=w259:errorcluster, "IsInPackedLibrary"=→"inlvlibp":bool)
            n97 = Close Reference(reference=w257, error in (no error)=w259) -> ()  [unwired: 1 out]
          }
        }
        n98 = feedback-in #2(w246) -> ()
      }
    }
    "Mode" <- w225
    "#Nodes" <- w227
    "#Elements In Queue" <- w226
    n99 = case shown="Default" w225 {
      tunnel: w233 -> [_ w238]
      tunnel: [_ w237] -> w231
      tunnel: [_ w236] -> w230
      tunnel: [_ w235] -> w224
      tunnel: [_ w234] -> w223
      frame "Not Exist", "Worker", "Chain" {
      }
      frame Default {
        n100 = in-place {
          in-place-border: [w240] -> w239
          n101 = in-place-dvr #3(w238) -> (w240:T12)  [unwired: 1 out]
          n102 = in-place-dvr #3(w240) -> ()  [unwired: 2 out]
        }
        n103 = Unbundle By Name(w239) -> ("RemoteMessge?"=w237:bool, "Initialized"=w236:enum16{"Initializing", "Ready", "Exiting"}, "Current State"=w235:string, "Remaing JKISM Queue"=w234:string)
      }
    }
    "RemoteMessge?" <- w231
    "Initialized" <- w230
    "Remaing States" <- w223
    "Current State" <- w224
    n104 = Wait (ms)(milliseconds to wait=u32 100) -> ()  [unwired: 1 out]
    n105 = local read "interStop"() -> (w232:bool)
  }
